vi "trace.payload_sent.vi"(6 "Headers":cluster{"header":string, "value":string}[](array[cluster]), 8 "dataflow error in":errorcluster, 9 "Request Body":string="<empty string>", 10 "Path":string) -> (0 "dataflow error out":errorcluster)   [LabVIEW 2020, in "Nominal Client.lvclass"]
uses:
  Nominal Client.lvclass
  <vilib>/Utility/libraryn.llb/Get File Extension.vi
  <vilib>/JDP Science/JDP Science Common Utilities/JDP Utility.lvlib
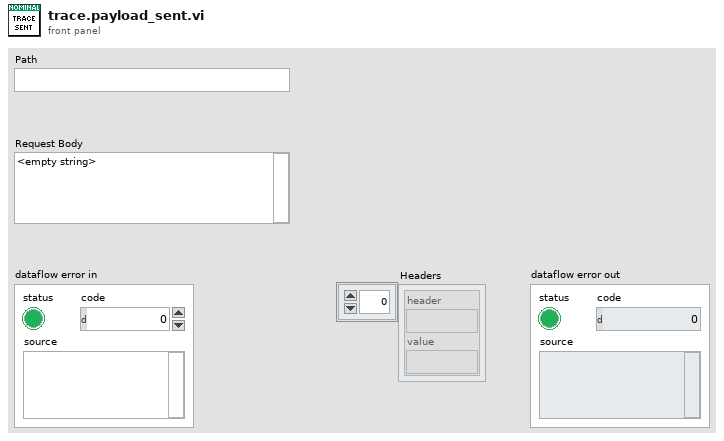
[diagram p1: front panel]
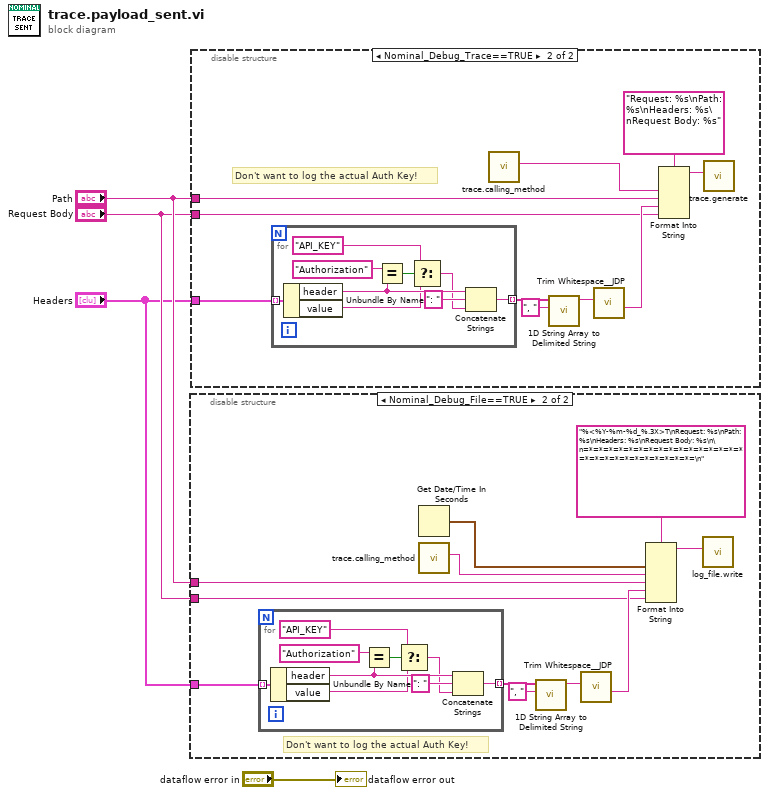
[diagram p0: block diagram]
diagram:
  n1 = disable-structure shown="Nominal_Debug_File==TRUE" {
    disable-tunnel: "Path" -> [_ w9]
    disable-tunnel: "Request Body" -> [_ w8]
    disable-tunnel: "Headers" -> [_ w7]
    frame condition #0 {
    }
    frame condition #1 (active) {
      # "Don't want to log the actual Auth Key!"
      n2 = for {
        tunnel: w7 -> [w24] mode=indexing
        tunnel: [w22] -> w14 mode=indexing
        n3 = Unbundle By Name(w24) -> ("header"=w20:string, "value"=w18:string)
        n4 = Equal?(x="Authorization", y=w20) -> (x = y?=w19:bool)
        n5 = Select(t="API_KEY", s=w19, f=w18) -> (s? t:f=w17:string)
        n6 = Concatenate Strings(w20, ": " ("string"), w17) -> (w22:string)
      }
      n7 = Get Date/Time In Seconds() -> (seconds since 1Jan1904=w5:timestamp)
      n8 = call "trace.calling_method.vi"() -> ("Calling Method Name"=w10:string)  [unwired: 11 in]
      n9 = call <vilib>:"1D String Array to Delimited String.vi"("delimiter"=", ", "string array"=w14) -> ("delimited string"=w12:string)  [unwired: 9 in]
      n10 = call <vilib>:"Trim Whitespace__JDP.vi"("String in"=w12) -> ("String out"=w11:string)  [unwired: 6 in]
      n11 = Format Into String(format string="%<%Y-%m-%d_%.3X>T\nRequest: %s\nPath: %s\nHeaders: %s\nRequest Body: %s\n\n=*=*=*=*=*=*=*=*=*=*=*=*=*=*=*=*=*=*=*=*=*=*=*=*=*=*=*=\n", w5, w10, w9, w11, w8) -> (resulting string=w6:string)  [unwired: 2 in, 1 out]
      n12 = call "log_file.write.vi"("trace string"=w6) -> ()  [unwired: 11 in]
    }
  }
  n13 = disable-structure shown="Nominal_Debug_Trace==TRUE" {
    disable-tunnel: "Path" -> [_ w27]
    disable-tunnel: "Request Body" -> [_ w25]
    disable-tunnel: "Headers" -> [_ w34]
    frame condition #0 {
    }
    frame condition #1 (active) {
      # "Don't want to log the actual Auth Key!"
      n14 = for {
        tunnel: w34 -> [w43] mode=indexing
        tunnel: [w41] -> w32 mode=indexing
        n15 = Unbundle By Name(w43) -> ("header"=w39:string, "value"=w37:string)
        n16 = Equal?(x="Authorization", y=w39) -> (x = y?=w38:bool)
        n17 = Select(t="API_KEY", s=w38, f=w37) -> (s? t:f=w36:string)
        n18 = Concatenate Strings(w39, ": " ("string"), w36) -> (w41:string)
      }
      n19 = call "trace.calling_method.vi"() -> ("Calling Method Name"=w28:string)  [unwired: 11 in]
      n20 = call <vilib>:"1D String Array to Delimited String.vi"("delimiter"=", ", "string array"=w32) -> ("delimited string"=w30:string)  [unwired: 9 in]
      n21 = call <vilib>:"Trim Whitespace__JDP.vi"("String in"=w30) -> ("String out"=w29:string)  [unwired: 6 in]
      n22 = Format Into String(format string="Request: %s\nPath: %s\nHeaders: %s\nRequest Body: %s", w28, w27, w29, w25) -> (resulting string=w26:string)  [unwired: 2 in, 1 out]
      n23 = call "trace.generate.vi"("trace string"=w26) -> ()  [unwired: 11 in]
    }
  }
  "dataflow error out" <- "dataflow error in"
